vi "initialization.vi"(9 "软件版本":refnum<vi>, 10 "updateconfiguration":refnum<vi>) -> ()   [LabVIEW 2016, in "数据传输系统-02.lvlib"]
uses:
  <vilib>/Utility/config.llb/Read Key (String).vi
  <vilib>/Utility/config.llb/NI_LVConfig.lvlib
panel:
  in  "参数数值":T1={"CODMn"=TRUE, "CODCr"=TRUE, "DO"=TRUE, "铜"=TRUE, "PH"=TRUE, "氨氮"=TRUE, "比电导率"=TRUE, "水温"=TRUE, "COD"=TRUE, "浊度"=TRUE, "总氮"=TRUE, "总磷"=TRUE, "叶绿素a"=TRUE, "藻密度"=TRUE, "水位"=TRUE, "流速"=TRUE, "方向"=TRUE, "瞬时流量"=TRUE, "累积流量"=TRUE, "正累积流量"=TRUE, "负累积流量"=TRUE, "亚硝氮"=TRUE, "硫化物"=TRUE, "ORP"=TRUE, "铅"=TRUE, "镉"=TRUE, "锌"=TRUE, "镍"=TRUE, "锰"=TRUE, "汞"=TRUE, "气温"=TRUE, "气压"=TRUE, "风速"=TRUE, "风向"=TRUE, "空气温度"=TRUE, "相对湿度"=TRUE, "分钟雨量"=TRUE, "小时雨量"=TRUE, "日雨量"=TRUE, "累积雨量"=TRUE, "盐度"=TRUE, "磷酸盐"=TRUE, "硝氮"=TRUE, "氟化物"=TRUE, "挥发酚"=TRUE, "氯化物"=TRUE, "蓝绿藻"=TRUE, "余氯"=TRUE, "综合生物毒性"=TRUE, "艏向"=TRUE, "横摇"=TRUE, "纵摇"=TRUE, "分层标志"=TRUE, "层状态1"=TRUE, "层状态2"=TRUE, "水平平均流速"=TRUE, "流向"=TRUE, "北向流速分量"=TRUE, "东向流速分量"=TRUE, "垂直流速分量"=TRUE, "最大波高"=TRUE, "最大波周期"=TRUE, "1/10波高"=TRUE, "1/10波周期"=TRUE, "有效波高"=TRUE, "有效波周期"=TRUE, "平均波高"=TRUE, "平均波周期"=TRUE, "波向"=TRUE, "波个数"=TRUE, "水深"=TRUE, "X轴流速"=TRUE, "Y轴流速"=TRUE, "信号强度"=TRUE, "电压"=TRUE, "悬浮物"=TRUE}
  out "配置表格":string[][](table)
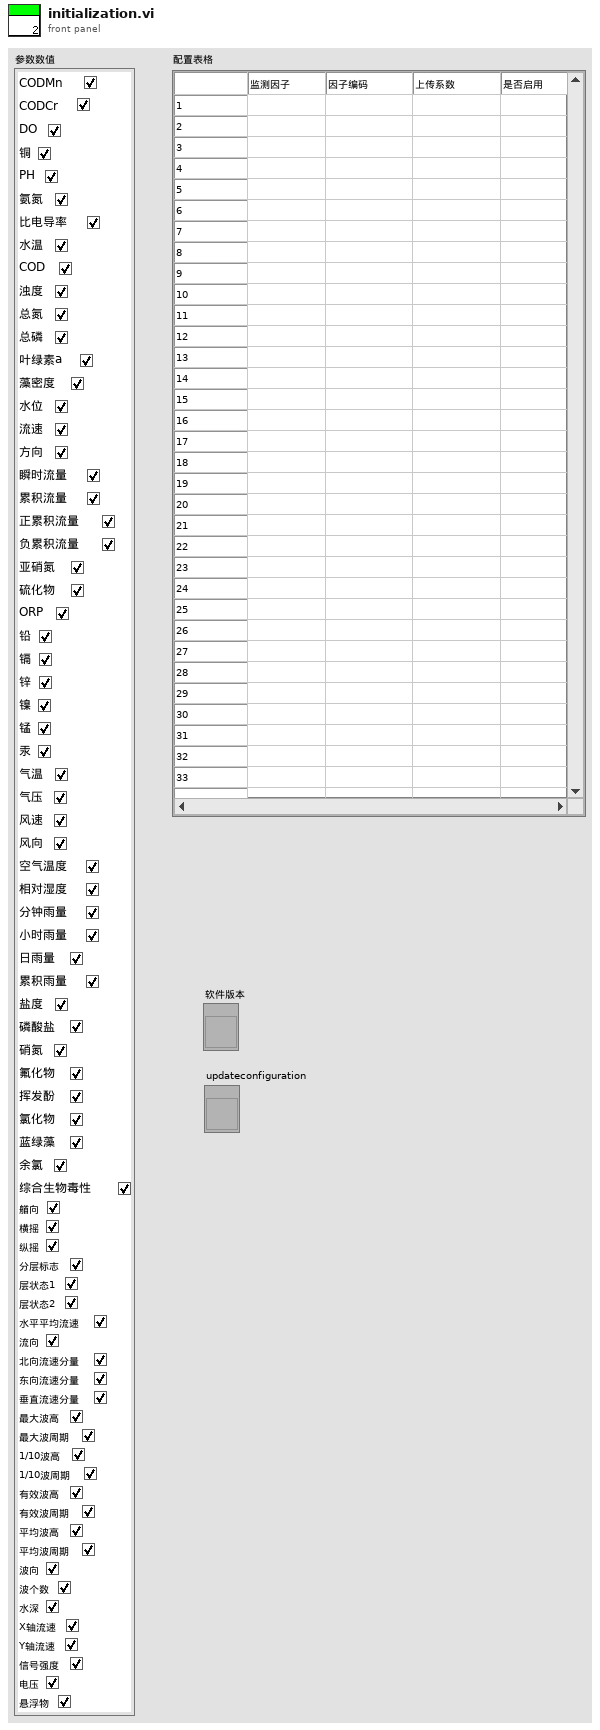
[diagram p1: front panel]
types:
  T1 = cluster{"CODMn":bool, "CODCr":bool, "DO":bool, "铜":bool, "PH":bool, "氨氮":bool, "比电导率":bool, "水温":bool, "COD":bool, "浊度":bool, "总氮":bool, "总磷":bool, "叶绿素a":bool, "藻密度":bool, "水位":bool, "流速":bool, "方向":bool, "瞬时流量":bool, "累积流量":bool, "正累积流量":bool, "负累积流量":bool, "亚硝氮":bool, "硫化物":bool, "ORP":bool, "铅":bool, "镉":bool, "锌":bool, "镍":bool, "锰":bool, "汞":bool, "气温":bool, "气压":bool, "风速":bool, "风向":bool, "空气温度":bool, "相对湿度":bool, "分钟雨量":bool, "小时雨量":bool, "日雨量":bool, "累积雨量":bool, "盐度":bool, "磷酸盐":bool, "硝氮":bool, "氟化物":bool, "挥发酚":bool, "氯化物":bool, "蓝绿藻":bool, "余氯":bool, "综合生物毒性":bool, "艏向":bool, "横摇":bool, "纵摇":bool, "分层标志":bool, "层状态1":bool, "层状态2":bool, "水平平均流速":bool, "流向":bool, "北向流速分量":bool, "东向流速分量":bool, "垂直流速分量":bool, "最大波高":bool, "最大波周期":bool, "1/10波高":bool, "1/10波周期":bool, "有效波高":bool, "有效波周期":bool, "平均波高":bool, "平均波周期":bool, "波向":bool, "波个数":bool, "水深":bool, "X轴流速":bool, "Y轴流速":bool, "信号强度":bool, "电压":bool, "悬浮物":bool}
  T2 = cluster{"setini":string, "sysini":string, "hechaini":string, "actualwrite":string, "actualread":string, "datasent":string, "反控命令信息队列":string, "反控与仪器交互":string}
  T3 = cluster{"CODMn":string, "CODCr":string, "DO":string, "铜":string, "PH":string, "氨氮":string, "比电导率":string, "水温":string, "COD":string, "浊度":string, "总氮":string, "总磷":string, "叶绿素a":string, "藻密度":string, "水位":string, "流速":string, "方向":string, "瞬时流量":string, "累积流量":string, "正累积流量":string, "负累积流量":string, "亚硝酸盐":string, "硫化物":string, "ORP":string, "铅":string, "镉":string, "锌":string, "镍":string, "锰":string, "汞":string, "气温":string, "气压":string, "风速":string, "风向":string, "空气温度":string, "相对湿度":string, "分钟雨量":string, "小时雨量":string, "日雨量":string, "累积雨量":string, "盐度":string, "磷酸盐":string, "硝氮":string, "氟化物":string, "挥发酚":string, "氯化物":string, "蓝绿藻":string, "余氯":string, "综合生物毒性":string, "艏向":string, "横摇":string, "纵摇":string, "分层标志":string, "层状态1":string, "层状态2":string, "水平平均流速":string, "流向":string, "北向流速分量":string, "东向流速分量":string, "垂直流速分量":string, "最大波高":string, "最大波周期":string, "1/10波高":string, "1/10波周期":string, "有效波高":string, "有效波周期":string, "平均波高":string, "平均波周期":string, "波向":string, "波个数":string, "水深":string, "X轴流速":string, "Y轴流速":string, "信号强度":string, "电压":string, "悬浮物":string}
  T4 = cluster{"主机":string, "用户":string, "密码":string, "远程路径":string, "下载文件名":string, "软件版本":string}
  T5 = typedef "NI_LVConfig.lvlib/Config Data RefNum.ctl" = refnum<k1>
  T6 = cluster{"子数组[0]":string, "子数组[1]":string, "子数组[2]":string, "子数组[3]":string, "子数组[4]":string, "子数组[5]":string, "子数组[6]":string, "子数组[7]":string, "子数组[8]":string, "子数组[9]":string, "子数组[10]":string, "子数组[11]":string, "子数组[12]":string, "子数组[13]":string, "子数组[14]":string, "子数组[15]":string, "子数组[16]":string, "子数组[17]":string, "子数组[18]":string, "子数组[19]":string, "子数组[20]":string, "子数组[21]":string, "子数组[22]":string, "子数组[23]":string, "子数组[24]":string, "子数组[25]":string, "子数组[26]":string, "子数组[27]":string, "子数组[28]":string, "子数组[29]":string, "子数组[30]":string, "子数组[31]":string, "子数组[32]":string, "子数组[33]":string, "子数组[34]":string, "子数组[35]":string, "子数组[36]":string, "子数组[37]":string, "子数组[38]":string, "子数组[39]":string, "子数组[40]":string, "子数组[41]":string, "子数组[42]":string, "子数组[43]":string, "子数组[44]":string, "子数组[45]":string, "子数组[46]":string, "子数组[47]":string, "子数组[48]":string, "子数组[49]":string, "子数组[50]":string, "子数组[51]":string, "子数组[52]":string, "子数组[53]":string, "子数组[54]":string, "子数组[55]":string, "子数组[56]":string, "子数组[57]":string, "子数组[58]":string, "子数组[59]":string, "子数组[60]":string, "子数组[61]":string, "子数组[62]":string, "子数组[63]":string, "子数组[64]":string, "子数组[65]":string, "子数组[66]":string, "子数组[67]":string, "子数组[68]":string, "子数组[69]":string, "子数组[70]":string, "子数组[71]":string, "子数组[72]":string, "子数组[73]":string, "子数组[74]":string, "子数组[75]":string}
  T7 = cluster{"[0]":string, "[1]":string, "[2]":string, "[3]":string, "[4]":string, "[5]":string, "[6]":string, "[7]":string, "[8]":string, "[9]":string, "[10]":string, "[11]":string, "[12]":string, "[13]":string, "[14]":string, "[15]":string, "[16]":string, "[17]":string, "[18]":string, "[19]":string, "[20]":string, "[21]":string, "[22]":string, "[23]":string, "[24]":string, "[25]":string, "[26]":string, "[27]":string, "[28]":string, "[29]":string, "[30]":string, "[31]":string, "[32]":string, "[33]":string, "[34]":string, "[35]":string, "[36]":string, "[37]":string, "[38]":string, "[39]":string, "[40]":string, "[41]":string, "[42]":string, "[43]":string, "[44]":string, "[45]":string, "[46]":string, "[47]":string, "[48]":string, "[49]":string, "[50]":string, "[51]":string, "[52]":string, "[53]":string, "[54]":string, "[55]":string, "[56]":string, "[57]":string, "[58]":string, "[59]":string, "[60]":string, "[61]":string, "[62]":string, "[63]":string, "[64]":string, "[65]":string, "[66]":string, "[67]":string, "[68]":string, "[69]":string, "[70]":string, "[71]":string, "[72]":string, "[73]":string, "[74]":string, "[75]":string}
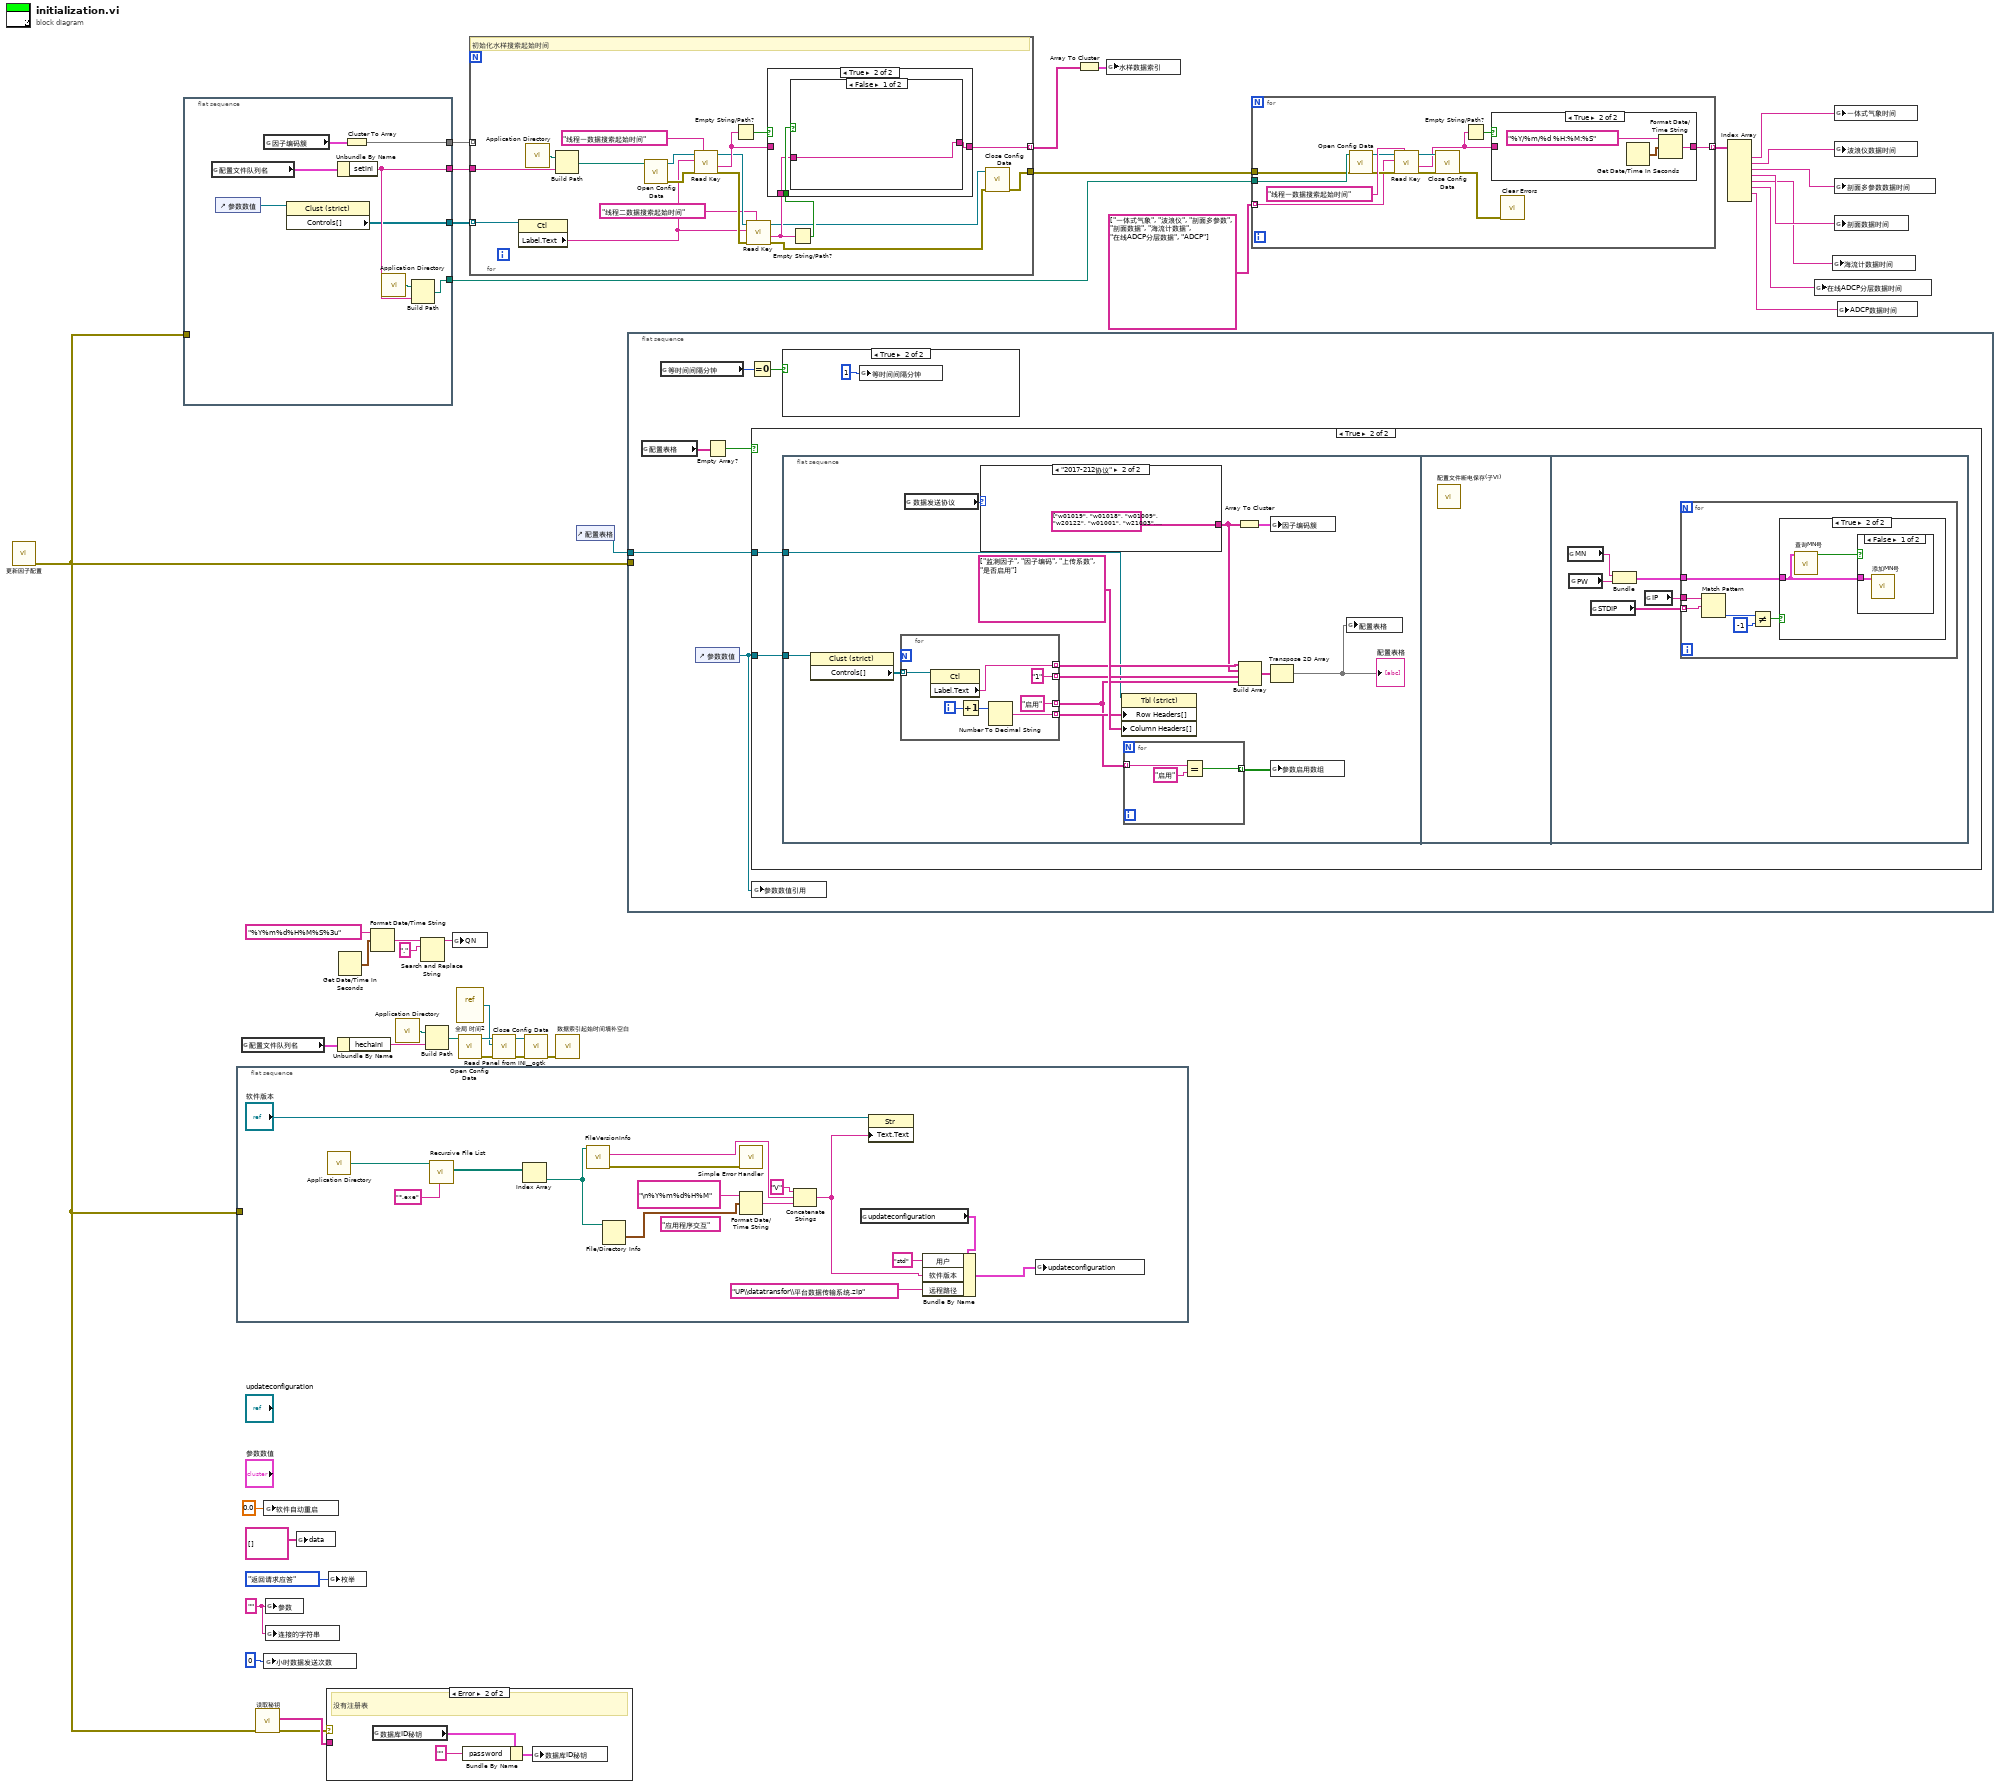
[diagram p0: block diagram]
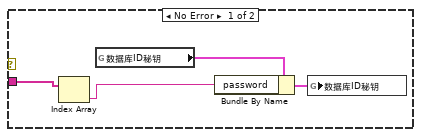
[diagram p2: hidden frame]
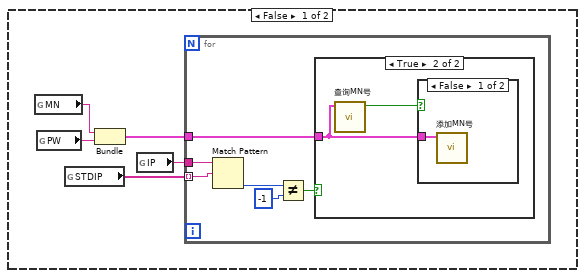
[diagram p4: hidden frame]
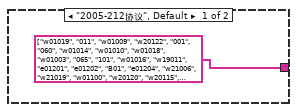
[diagram p7: hidden frame]
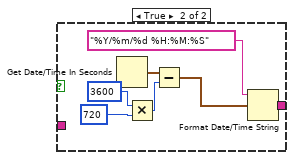
[diagram p12: hidden frame]
diagram:
  w16 = "" ("参数")
  n1 = call "更新因子配置.vi"() -> ("error out"=w1:errorcluster)  [unwired: 11 in]
  n2 = flat-sequence {
    tunnel: [w48] -> w38
    tunnel: [w46] -> w35
    tunnel: [w44] -> w32
    tunnel: [w42] -> w10
    tunnel: w1 -> [_]
    frame #0 {
      n3 = global read "全局1.vi" "配置文件队列名"() -> (w43:T2)
      n4 = control-ref of="参数数值"() -> (w41:refnum<vi>)
      n5 = global read "断电保存全局.vi" "因子编码簇"() -> (w47:T3)
      n6 = property class="Clust (strict)"(reference=w41) -> ("Controls[]"=w42:refnum<vi>[])  [unwired: 1 in, 2 out]
      n7 = Unbundle By Name(w43) -> ("setini"=w48:string)
      n8 = Cluster To Array(cluster=w47) -> (array=w44:string[])
      n9 = call <vilib>:"Application Directory.vi"() -> ("Application Directory"=w45:path)
      n10 = Build Path(base path=w45, name or relative path=w48) -> (appended path=w46:path)
    }
  }
  n11 = flat-sequence {
    tunnel: w1 -> [_]
    frame #0 {
      (unwired) "应用程序交互" ("section")
      n12 = call <vilib>:"Application Directory.vi"() -> ("Application Directory"=w62:path)
      n13 = call <vilib>:"Recursive File List.vi"("pattern"="*.exe", "Folder Path"=w62) -> ("All Files in Dir"=w56:path[])  [unwired: 5 in, 4 out]
      n14 = Index Array(array=w56) -> (element=w57:path)  [unwired: 1 in]
      n15 = call <vilib>:"FileVersionInfo.vi"("Application Path in"=w57) -> ("error out"=w63:errorcluster, "File Version Info"=w64:string)  [unwired: 7 in, 2 out]
      n16 = File/Directory Info(path=w57) -> (last mod=w58:timestamp)  [unwired: 1 in, 6 out]
      n17 = call <vilib>:"Simple Error Handler.vi"("error in (no error)"=w63) -> ()  [unwired: 4 in, 5 out]
      n18 = Format Date/Time String(time format string (%c)="\n%Y%m%d%H%M" ("时间格式字符串(%c)"), seconds (now)=w58) -> (date/time string=w61:string)  [unwired: 1 in]
      n19 = Concatenate Strings("V" ("字符串"), w64, w61) -> (w53:string)
      n20 = global read "断电保存全局.vi" "updateconfiguration"() -> (w50:T4)
      n21 = property class="Str"(reference="软件版本", "Text.Text"=w53) -> ()  [unwired: 1 in, 2 out]
      n22 = Bundle By Name(cluster=w50, "用户"="std", "软件版本"=w53, "远程路径"="UP\\datatransfor\\平台数据传输系统.zip") -> (w52:T4)
      n23 = global write "断电保存全局.vi" "updateconfiguration"(w52) -> ()
    }
  }
  n24 = global read "全局1.vi" "配置文件队列名"() -> (w13:T2)
  n25 = call "读取秘钥.vi"("error in (no error)"=w1) -> ("error out"=w11:errorcluster, "值"=w12:string[])  [unwired: 8 in, 1 out]
  n26 = global write "全局1.vi" "软件自动重启"(0.0 ("软件自动重启")) -> ()
  n27 = global write "全局 小时数据发送次数.vi" "小时数据发送次数"(0 ("数值")) -> ()
  n28 = global write "全局 实时数据参数.vi" "参数"(w16) -> ()
  n29 = global write "全局 实时数据参数.vi" "连接的字符串"(w16) -> ()
  n30 = global write "全局 实时数据参数.vi" "data"(string[][] [] ("data")) -> ()
  n31 = case shown="Error" w11 {
    tunnel: w12 -> [w68 _]
    frame No Error {
      n32 = Index Array(array=w68) -> (element=w65:string)  [unwired: 1 in]
      n33 = global read "外部交互全局.vi" "数据库ID秘钥"() -> (w66:cluster{"userID":string, "password":string})
      n34 = Bundle By Name(cluster=w66, "password"=w65) -> (w67:cluster{"userID":string, "password":string})
      n35 = global write "外部交互全局.vi" "数据库ID秘钥"(w67) -> ()
    }
    frame Error {
      # "没有注册表"
      n36 = global read "外部交互全局.vi" "数据库ID秘钥"() -> (w69:cluster{"userID":string, "password":string})
      n37 = Bundle By Name(cluster=w69, "password"="") -> (w70:cluster{"userID":string, "password":string})
      n38 = global write "外部交互全局.vi" "数据库ID秘钥"(w70) -> ()
    }
  }
  n39 = global write "全局1.vi" "枚举"(enum16{"返回请求应答", "上传数据", "返回执行结果"}."返回请求应答" ("枚举")) -> ()
  n40 = Unbundle By Name(w13) -> ("hechaini"=w39:string)
  n41 = Get Date/Time In Seconds() -> (seconds since 1Jan1904=w20:timestamp)
  n42 = Format Date/Time String(time format string (%c)="%Y%m%d%H%M%S%3u" ("时间格式字符串(%c)"), seconds (now)=w20) -> (date/time string=w21:string)  [unwired: 1 in]
  n43 = call <vilib>:"Application Directory.vi"() -> ("Application Directory"=w25:path)
  n44 = Search and Replace String(input string=w21, search string="." ("搜索字符串")) -> (result string=w23:string)  [unwired: 6 in, 3 out]
  n45 = Build Path(base path=w25, name or relative path=w39) -> (appended path=w24:path)
  n46 = global write "全局1.vi" "QN"(w23) -> ()
  n47 = vi-ref "全局 时间2.vi"() -> (w27:refnum<vi>)
  n48 = call <vilib>:"Open Config Data.vi"("configuration file path"=w24) -> ("error out"=w29:errorcluster, "refnum"=w28:T5)  [unwired: 8 in, 1 out]
  n49 = for {
    tunnel: w32 -> [_] mode=indexing
    tunnel: [w83] -> w33 mode=indexing
    tunnel: [w82] -> w36
    tunnel: w38 -> [w81]
    tunnel: w10 -> [w80] mode=indexing
    # "初始化水样搜索起始时间"
    n50 = property class="Ctl"(reference=w80) -> ("Label.Text"=w72:string)  [unwired: 1 in, 2 out]
    n51 = call <vilib>:"Application Directory.vi"() -> ("Application Directory"=w90:path)
    n52 = Build Path(base path=w90, name or relative path=w81) -> (appended path=w89:path)
    n53 = call <vilib>:"Open Config Data.vi"("configuration file path"=w89) -> ("error out"=w87:errorcluster, "refnum"=w88:T5)  [unwired: 8 in, 1 out]
    n54 = call-poly <vilib>:"Read Key.vi"("section"="线程一数据搜索起始时间", "error in (no error)"=w87, "key"=w72, "refnum"=w88) -> ("error out"=w78:errorcluster, "value"=w84:string, "refnum out"=w79:T5)  [unwired: 4 in, 1 out]
    n55 = Empty String/Path?(string/path=w84) -> (empty?=w85:bool)
    n56 = call-poly <vilib>:"Read Key.vi"("section"="线程二数据搜索起始时间", "error in (no error)"=w78, "key"=w72, "refnum"=w79) -> ("error out"=w73:errorcluster, "value"=w75:string, "refnum out"=w74:T5)  [unwired: 4 in, 1 out]
    n57 = Empty String/Path?(string/path=w75) -> (empty?=w76:bool)
    n58 = case shown="True" w85 {
      tunnel: [w91 w94] -> w83
      tunnel: w84 -> [w91 _]
      tunnel: w76 -> [_ w93]
      tunnel: w75 -> [_ w92]
      frame False {
      }
      frame True {
        n59 = case shown="False" w93 {
          tunnel: [w95 w101] -> w94
          tunnel: w92 -> [w95 _]
          frame False {
          }
          frame True {
            n60 = Get Date/Time In Seconds() -> (seconds since 1Jan1904=w100:timestamp)
            n61 = Multiply(x=3600, y=720) -> (x*y=w97:i32)
            n62 = Subtract(x=w100, y=w97) -> (x-y=w96:timestamp)
            n63 = Format Date/Time String(time format string (%c)="%Y/%m/%d %H:%M:%S" ("时间格式字符串(%c)"), seconds (now)=w96) -> (date/time string=w101:string)  [unwired: 1 in]
          }
        }
      }
    }
    n64 = call <vilib>:"Close Config Data.vi"("error in (no error)"=w73, "refnum"=w74) -> ("error out"=w82:errorcluster)  [unwired: 8 in, 1 out]
  }
  n65 = call <userlib>:"Read Panel from INI__ogtk.vi"("error in (no error)"=w29, "VI ref"=w27, "refnum"=w28) -> ("error out"=w30:errorcluster, "refnum out"=w26:T5)  [unwired: 7 in]
  n66 = call <vilib>:"Close Config Data.vi"("error in (no error)"=w30, "refnum"=w26) -> ("error out"=w31:errorcluster)  [unwired: 8 in, 1 out]
  n67 = call "数据索引起始时间填补空白.vi"("error in (no error)"=w31) -> ()  [unwired: 10 in, 1 out]
  n68 = control-ref of="配置表格"() -> (w14:refnum<vi>)
  n69 = flat-sequence {
    tunnel: w1 -> [_]
    tunnel: w14 -> [w107]
    frame #0 {
      n70 = global read "断电保存全局.vi" "配置表格"() -> (w108:string[][])
      n71 = global read "断电保存全局.vi" "等时间间隔分钟"() -> (w104:i32)
      n72 = control-ref of="参数数值"() -> (w106:refnum<vi>)
      n73 = Empty Array?(array=w108) -> (empty?=w103:bool)
      n74 = Equal To 0?(x=w104) -> (x = 0?=w105:bool)
      n75 = case shown="True" w103 {
        tunnel: w107 -> [_ w125]
        tunnel: w106 -> [_ w124]
        frame False {
          n76 = global read "断电保存全局.vi" "MN"() -> (w114:string)
          n77 = global read "断电保存全局.vi" "PW"() -> (w113:string)
          n78 = global read "断电保存全局.vi" "STDIP"() -> (w111:string[])
          n79 = Bundle("MN"=w114, "PW"=w113) -> (w112:cluster{"MN":string, "PW":string})  [unwired: 1 in]
          n80 = global read "断电保存全局.vi" "IP"() -> (w110:string)
          n81 = for {
            tunnel: w111 -> [w120] mode=indexing
            tunnel: w110 -> [w119]
            tunnel: w112 -> [w115]
            n82 = Match Pattern(string=w119, regular expression=w120) -> (offset past match=w118:i32)  [unwired: 1 in, 3 out]
            n83 = Not Equal?(x=w118, y=-1) -> (x != y?=w116:bool)
            n84 = case shown="True" w116 {
              tunnel: w115 -> [_ w122]
              frame False {
              }
              frame True {
                n85 = call "查询MN号.vi"("簇"=w122) -> ("包含启动项"=w121:bool)  [unwired: 9 in, 1 out]
                n86 = case shown="False" w121 {
                  tunnel: w122 -> [w123 _]
                  frame False {
                    n87 = call "添加MN号.vi"("簇"=w123) -> ()  [unwired: 9 in, 2 out]
                  }
                  frame True {
                  }
                }
              }
            }
          }
        }
        frame True {
          n88 = flat-sequence {
            tunnel: w125 -> [w127]
            tunnel: w124 -> [w126]
            frame #0 {
              n89 = property on="属性节点" class="Clust (strict)"(reference=w126) -> ("Controls[]"=w135:refnum<vi>[])  [unwired: 1 in, 2 out]
              n90 = for {
                tunnel: w135 -> [w151] mode=indexing
                tunnel: [w150] -> w137 mode=indexing
                tunnel: [w148] -> w136 mode=indexing
                tunnel: ["1"] -> w130 mode=indexing
                tunnel: ["启用"] -> w129 mode=indexing
                i -> [w149]
                n91 = property class="Ctl"(reference=w151) -> ("Label.Text"=w150:string)  [unwired: 1 in, 2 out]
                n92 = Increment(x=w149) -> (x+1=w147:i32)
                n93 = Number To Decimal String(number=w147) -> (decimal integer string=w148:string)  [unwired: 1 in]
              }
              n94 = global read "断电保存全局.vi" "数据发送协议"() -> (w133:enum16{"2005-212协议", "2017-212协议"})
              n95 = case shown="\"2017-212协议\"" w133 {
                tunnel: [string[] ["w01019", "011", "w01009", "w20122", "001", "060", "w01014", "w01010", "w01018", "w01003", "065", "101", "w01016", "w19011", "e01201", "e01202", "B01", "e01204", "w21006", "w21019", "w01100", "w20120", "w20115", "w20123", "w20121", "w20124", "w20111", "a01001", "a01006", "a01007", "a01008", "w01002", "w21015", "w21007", "w21017", "w23002", "w21002", "w01022"] string[] ["w01019", "w01018", "w01009", "w20122", "w01001", "w21003", "w01014", "w01010", "w01018", "w01003", "w21001", "w21011", "w01016", "w19011", "e01201", "e01202", "e81205", "e01203", "e01204", "e81208", "e81209", "w21006", "w21019", "w01100", "w20120", "w20115", "w20123", "w20121", "w20124", "w20111", "a01001", "e01901", "e01301", "e01302", "e01001", "e01002", "e01303", "e013031", "e013032", "e013033", "w01002", "w21015", "w21007", "w21017", "w23002", "w21002", "w01022", "w21012", "w01023", "e81216", "e81217", "e81218", "e81220", "e81221", "e81222", "e81225", "e80015", "e81223", "e81224", "e81219", "e80001", "e80002", "e80003", "e80004", "e80005", "e80006", "e80007", "e80008", "e80009", "e80016", "e81231", "e81226", "e81227", "e81228", "e81215", "w01012"] ("子数组")] -> w131
                frame "2005-212协议", Default {
                }
                frame "2017-212协议" {
                }
              }
              n96 = property on="属性节点" class="Tbl (strict)"(reference=w127, "Row Headers[]"=w136, "Column Headers[]"=string[] ["监测因子", "因子编码", "上传系数", "是否启用"]) -> ()  [unwired: 1 in, 2 out]
              n97 = for {
                tunnel: w129 -> [w142] mode=indexing
                tunnel: [w140] -> w128 mode=indexing
                n98 = Equal?(x=w142, y="启用") -> (x = y?=w140:bool)
              }
              n99 = Array To Cluster(array=w131) -> (cluster=w132:T6)
              n100 = Build Array(w137, w131, w130, w129) -> (w139:string[][])
              n101 = global write "断电保存全局.vi" "因子编码簇"(w132) -> ()
              n102 = Transpose 2D Array(2D array=w139) -> (transposed array=w134:string[][])
              "配置表格" <- w134
              n103 = global write "断电保存全局.vi" "参数启用数组"(w128) -> ()
              n104 = global write "断电保存全局.vi" "配置表格"(w134) -> ()
            }
            frame #1 {
              n105 = call "配置文件断电保存(子VI).vi"() -> ()  [unwired: 12 in]
            }
            frame #2 {
              n106 = global read "断电保存全局.vi" "MN"() -> (w156:string)
              n107 = global read "断电保存全局.vi" "PW"() -> (w155:string)
              n108 = global read "断电保存全局.vi" "STDIP"() -> (w153:string[])
              n109 = Bundle("MN"=w156, "PW"=w155) -> (w154:cluster{"MN":string, "PW":string})  [unwired: 1 in]
              n110 = global read "断电保存全局.vi" "IP"() -> (w152:string)
              n111 = for {
                tunnel: w153 -> [w162] mode=indexing
                tunnel: w152 -> [w161]
                tunnel: w154 -> [w157]
                n112 = Match Pattern(string=w161, regular expression=w162) -> (offset past match=w160:i32)  [unwired: 1 in, 3 out]
                n113 = Not Equal?(x=w160, y=-1) -> (x != y?=w158:bool)
                n114 = case shown="True" w158 {
                  tunnel: w157 -> [_ w164]
                  frame False {
                  }
                  frame True {
                    n115 = call "查询MN号.vi"("簇"=w164) -> ("包含启动项"=w163:bool)  [unwired: 9 in, 1 out]
                    n116 = case shown="False" w163 {
                      tunnel: w164 -> [w165 _]
                      frame False {
                        n117 = call "添加MN号.vi"("簇"=w165) -> ()  [unwired: 9 in, 2 out]
                      }
                      frame True {
                      }
                    }
                  }
                }
              }
            }
          }
        }
      }
      n118 = global write "断电保存全局.vi" "参数数值引用"(w106) -> ()
      n119 = case shown="True" w105 {
        frame False {
        }
        frame True {
          n120 = global write "断电保存全局.vi" "等时间间隔分钟"(1 ("等时间间隔分钟")) -> ()
        }
      }
    }
  }
  n121 = Array To Cluster(array=w33) -> (cluster=w34:T7)
  n122 = global write "全局 水样时间.vi" "水样数据索引"(w34) -> ()
  n123 = for {
    tunnel: w35 -> [w177]
    tunnel: w36 -> [w176]
    tunnel: string[] ["一体式气象", "波浪仪", "剖面多参数", "剖面数据", "海流计数据", "在线ADCP分层数据", "ADCP"] -> [w168] mode=indexing
    tunnel: [w167] -> w40 mode=indexing
    n124 = call <vilib>:"Open Config Data.vi"("error in (no error)"=w176, "configuration file path"=w177) -> ("error out"=w173:errorcluster, "refnum"=w174:T5)  [unwired: 7 in, 1 out]
    n125 = call-poly <vilib>:"Read Key.vi"("section"="线程一数据搜索起始时间", "error in (no error)"=w173, "key"=w168, "refnum"=w174) -> ("error out"=w171:errorcluster, "value"=w170:string, "refnum out"=w172:T5)  [unwired: 4 in, 1 out]
    n126 = call <vilib>:"Close Config Data.vi"("error in (no error)"=w171, "refnum"=w172) -> ("error out"=w166:errorcluster)  [unwired: 8 in, 1 out]
    n127 = Empty String/Path?(string/path=w170) -> (empty?=w169:bool)
    n128 = case shown="True" w169 {
      tunnel: [w178 w179] -> w167
      tunnel: w170 -> [w178 _]
      frame False {
      }
      frame True {
        n129 = Get Date/Time In Seconds() -> (seconds since 1Jan1904=w181:timestamp)
        n130 = Format Date/Time String(time format string (%c)="%Y/%m/%d %H:%M:%S" ("时间格式字符串(%c)"), seconds (now)=w181) -> (date/time string=w179:string)  [unwired: 1 in]
      }
    }
    n131 = call <vilib>:"Clear Errors.vi"("error in (no error)"=w166) -> ()  [unwired: 5 in, 2 out]
  }
  n132 = Index Array(array=w40) -> (element #1=w7:string, element #2=w8:string, element #3=w6:string, element #4=w5:string, element #5=w4:string, element #6=w3:string, element #7=w2:string)  [unwired: 8 in, 1 out]
  n133 = global write "全局 水样时间.vi" "在线ADCP分层数据时间"(w3) -> ()
  n134 = global write "全局 水样时间.vi" "海流计数据时间"(w4) -> ()
  n135 = global write "全局 水样时间.vi" "一体式气象时间"(w7) -> ()
  n136 = global write "全局 水样时间.vi" "波浪仪数据时间"(w8) -> ()
  n137 = global write "全局 水样时间.vi" "剖面多参数数据时间"(w6) -> ()
  n138 = global write "全局 水样时间.vi" "剖面数据时间"(w5) -> ()
  n139 = global write "全局 水样时间.vi" "ADCP数据时间"(w2) -> ()
